vi "DriveUntilY.vi"(7 "Ultrasonic Stop":dbl, 8 "error in":errorcluster, 9 "y":dbl, 10 "x":dbl) -> (0 "error out":errorcluster)   [LabVIEW 2017]
uses:
  <vilib>/Rock Robotics/WPI/Ultrasonic/WPI_SonarMB1010AnalogRefNum Registry Get.vi
  Robot Global Data.vi
  <vilib>/Rock Robotics/WPI/Ultrasonic/WPI_SonarMB1010AnalogGetRange.vi
panel:
  # "DriveUntilY Autonomous Commands\nTeam 34 Rockets"
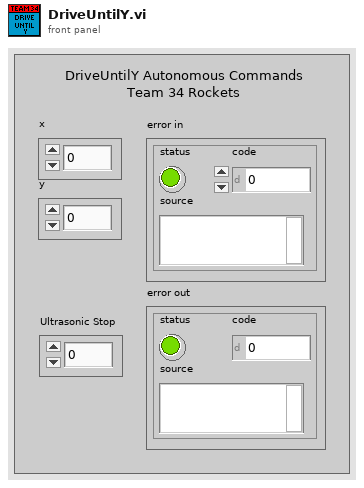
[diagram p1: front panel]
types:
  T1 = typedef "WPI_SonarMB1010AnalogDeviceRef.ctl" = cluster{"AIDeviceRef":T2, "Scaling factor (V/in)":dbl, "Average Bits":u8}
  T2 = typedef "WPI_AnalogChannelDevRef.ctl" = cluster{"DevStatus":errorcluster, "Analog Channel":T3}
  T3 = typedef "FPGA_AIChannel.ctl" = enum8{"AI 0", "AI 1", "AI 2", "AI 3", "AI MXP 0", "AI MXP 1", "AI MXP 2", "AI MXP 3", "Invalid"}
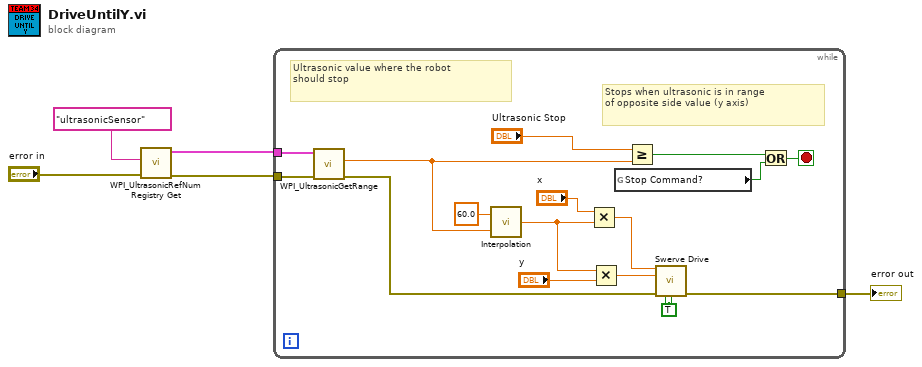
[diagram p0: block diagram]
diagram:
  n1 = call-poly <vilib>:"WPI_UltrasonicRefNum Registry Get.vi"("error in (no error)"="error in", "refnum name"="ultrasonicSensor") -> ("error out"=w1:errorcluster, "SonarMB1010AnalogDevRef"=w2:T1)  [unwired: 8 in]
  n2 = while {
    tunnel: w1 -> [w20]
    tunnel: w2 -> [w21]
    tunnel: [w16] -> w4
    stop <- w18 stop-if-true
    w15 = TRUE ("Autonomous?")
    # "Ultrasonic value where the robot\nshould stop"
    # "Stops when ultrasonic is in range\nof opposite side value (y axis)"
    n3 = call-poly <vilib>:"WPI_UltrasonicGetRange.vi"("error in"=w20, "SonarMB1010AnalogDevRef"=w21) -> ("error out"=w17:errorcluster, "Distance"=w8:dbl)  [unwired: 7 in, 1 out]
    n4 = call "Interpolation.vi"("Current Ultrasonic Distance"=w8, "Start Distance"=60.0) -> ("Motor Output"=w6:dbl)
    n5 = Multiply(x="x", y=w6) -> (x*y=w11:dbl)
    n6 = Multiply(x=w6, y="y") -> (x*y=w9:dbl)
    n7 = global read "Robot Global Data.vi" "Stop Command?"() -> (w19:bool)
    n8 = Greater Or Equal?(x="Ultrasonic Stop", y=w8) -> (x >= y?=w14:bool)
    n9 = call "Swerve Drive.vi"("X"=w11, "Y"=w9, "Error In"=w17, "Robot Centric?"=w15, "Autonomous?"=w15) -> ("Error Out"=w16:errorcluster)  [unwired: 6 in, 4 out]
    n10 = Or(x=w14, y=w19) -> (x .or. y?=w18:bool)
  }
  "error out" <- w4
